vi "LABWAD.vi"() -> ()   [LabVIEW 2017]
uses:
  SubVIs/WAD_MainCluster.ctl
  SubVIs/TextureList.ctl
  SubVIs/PatchList.ctl
  SubVIs/Lumps.ctl
  SubVIs/PLAYPAL.ctl
  Fire/Spread Fire.vi
  <vilib>/picture/picture.llb/Draw 8-Bit Pixmap.vi
  <userlib>/_OpenG.lib/array/array.llb/Filter 1D Array (String)__ogtk.vi
  <userlib>/_OpenG.lib/array/array.llb/Filter 1D Array with Scalar (String)__ogtk.vi
  <vilib>/regexp/Match Regular Expression.xnode
panel:
  out "2D Picture":picture
  in  "File Structure":string[](tree)
  out "Demonic Intensity Graph":i32[][](graph)
  # "Overview: Demonstrates how to read WAD files from original DOOM games.\nRequirements: LabVIEW Full Development System 2017 or compatible\nInstructions:\n1. Run this VI.\n2. Select a .wad file using the File > Open WAD File menu.\n3. Click on different items in the tree view to display them.\n4. Export the displayed image as PNG via drop-down menu on picture, or\n    select and export multiple items from the tree list via drop-down menu.\n5. Quit by using the File > Quit menu."
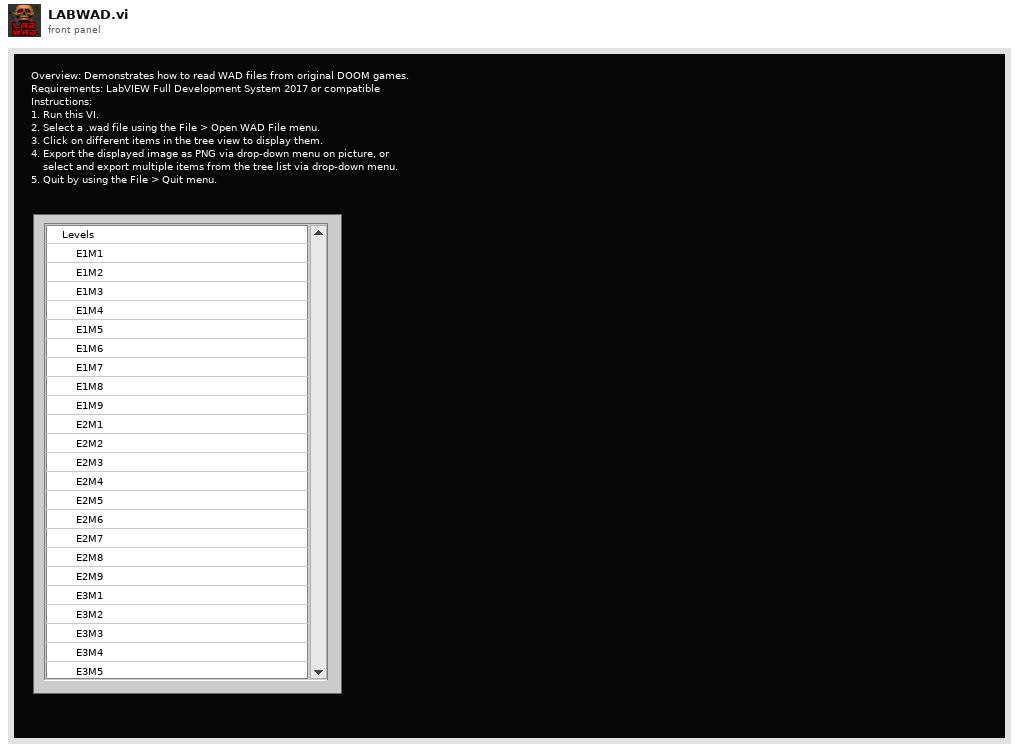
[diagram p1: front panel]
types:
  T1 = typedef "WAD_MainCluster.ctl" = cluster{"WAD file path":path, "WAD as U8 Array":u8[], "WAD Tree":refnum<vi>, "Palette":u32[], "TextureList":T2[], "PNAMES":string[], "Image Array":i16[][], "2D Picture":picture, "Lumps List":string[], "Lumps Array":T4[], "Textures Names":string[], "Image Mask":i16[][], "S_START Index":i32}
  T2 = typedef "TextureList.ctl" = cluster{"Name":string, "flags":u16, "masked":i16, "width":i16, "height":i16, "columndirectory":u32, "patchcount":i16, "PatchList":T3[]}
  T3 = typedef "PatchList.ctl" = cluster{"originx":i16, "originy":i16, "patch":i16}
  T4 = typedef "Lumps.ctl" = cluster{"offData":i32, "lenData":i32, "name":string}
  T5 = typedef "imagedata.ctl" = cluster{"image type":i32, "image depth":i32, "image":u8[], "mask":u8[], "colors":u32[], "Rectangle":cluster{"left":i16, "top":i16, "right":i16, "bottom":i16}}
  T6 = typedef "PatchHeader.ctl" = cluster{"Width":u16, "Height":u16, "XOffset":i16, "YOffset":i16}
  T7 = typedef "PLAYPAL.ctl" = u32[]
  T8 = typedef "LVBoundsTypeDef.ctl" = cluster{"Width":u32, "Height":u32}
  T9 = cluster{"ItemTag":string, "Navigate Tree:Get Path":string[][]}
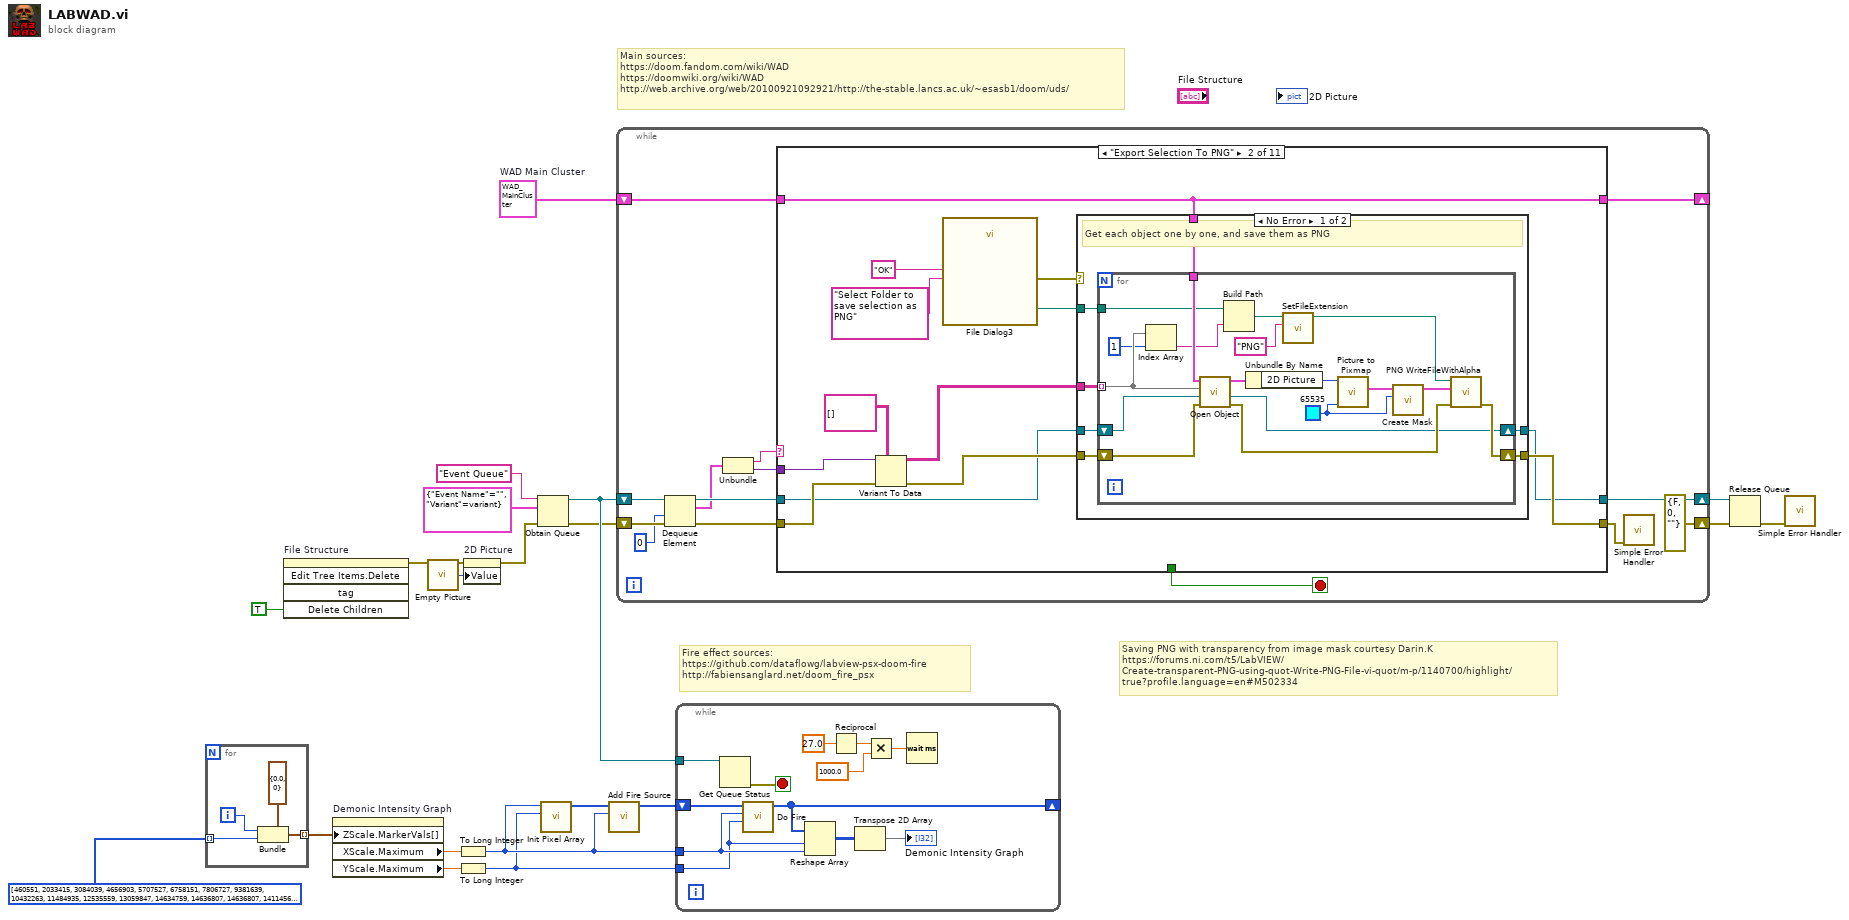
[diagram p0: block diagram]
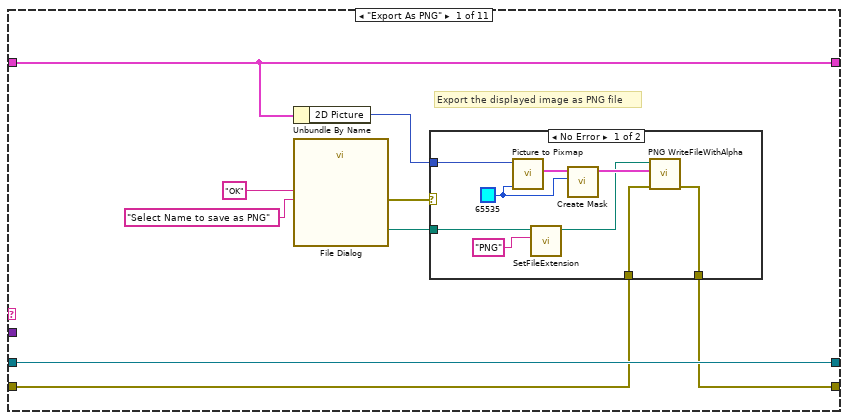
[diagram p2: hidden frame]
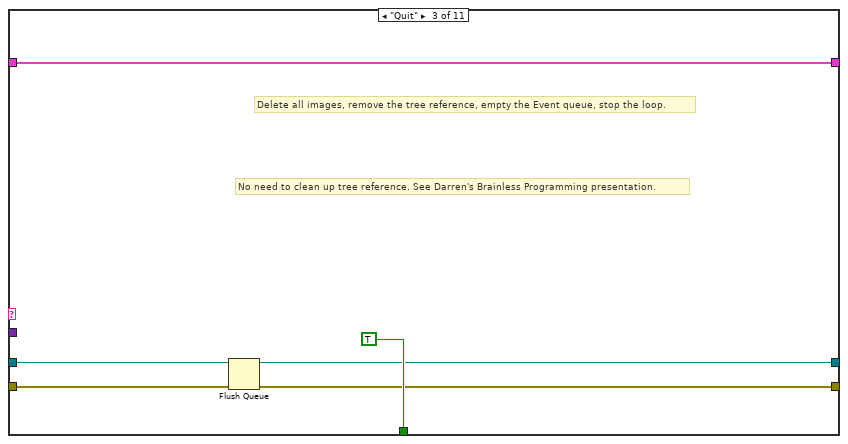
[diagram p5: hidden frame]
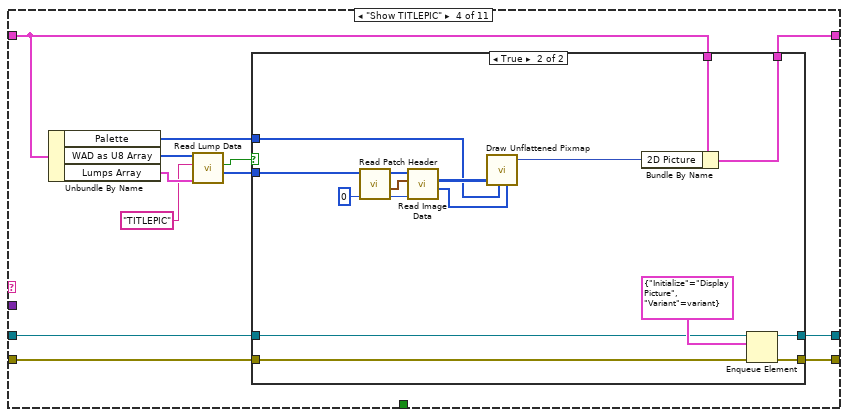
[diagram p6: hidden frame]
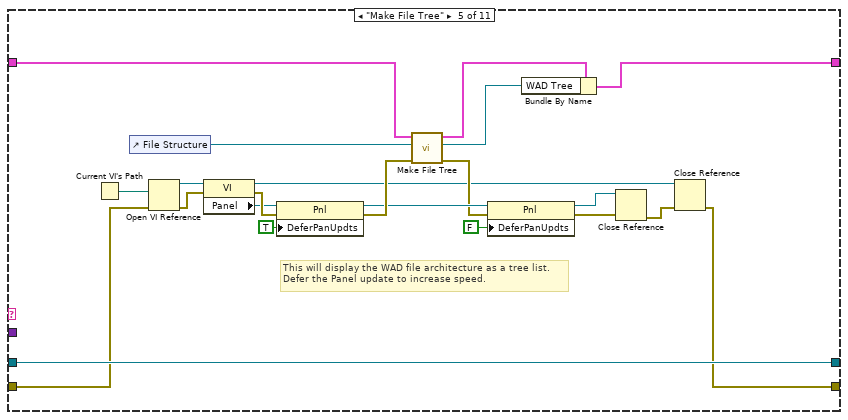
[diagram p8: hidden frame]
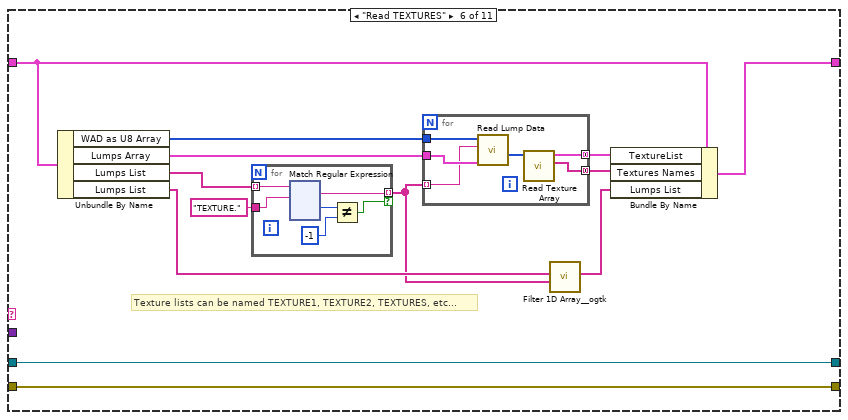
[diagram p9: hidden frame]
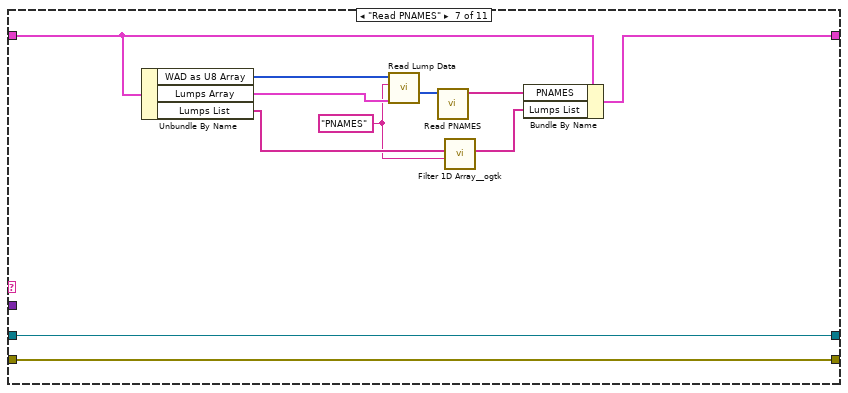
[diagram p10: hidden frame]
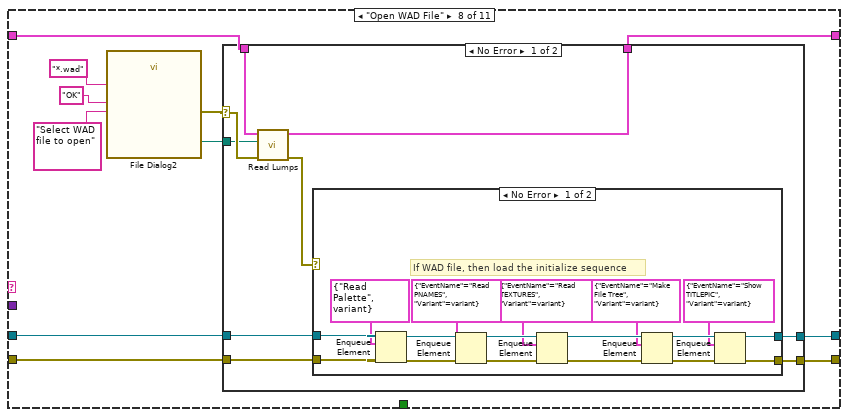
[diagram p11: hidden frame]
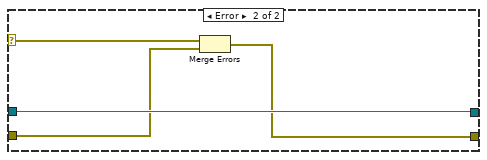
[diagram p12: hidden frame]
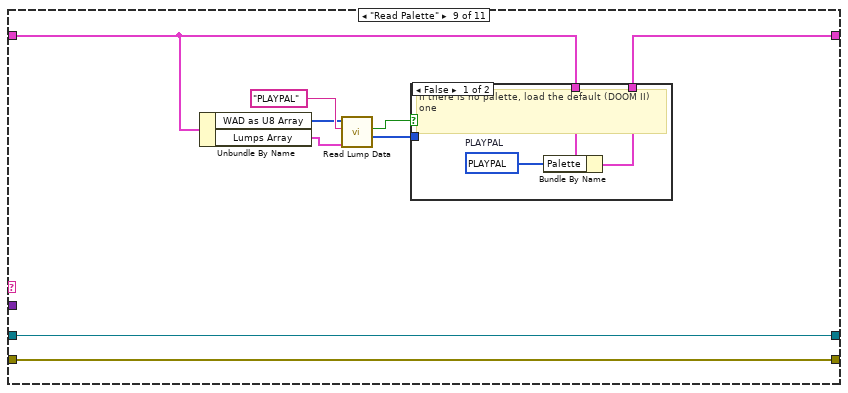
[diagram p14: hidden frame]
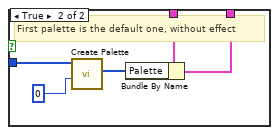
[diagram p15: hidden frame]
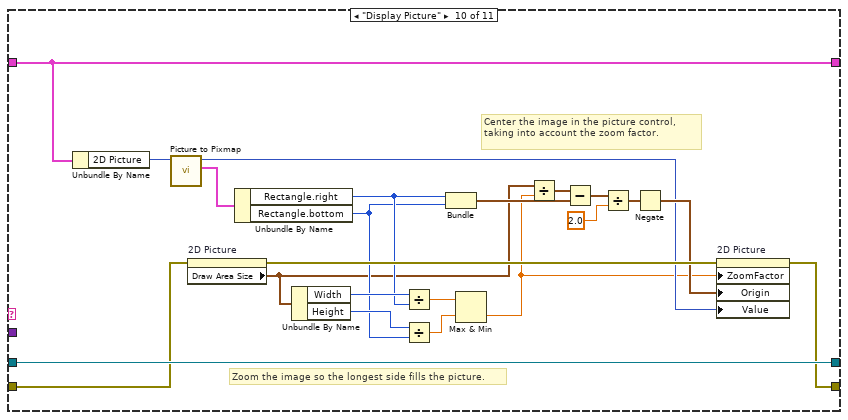
[diagram p16: hidden frame]
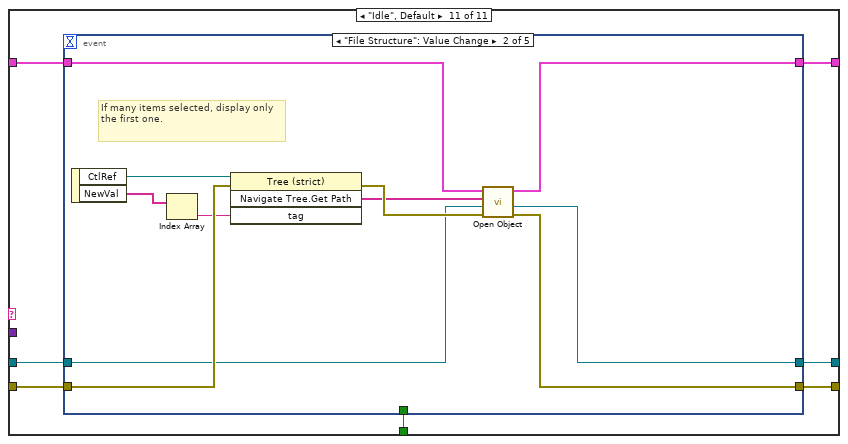
[diagram p17: hidden frame]
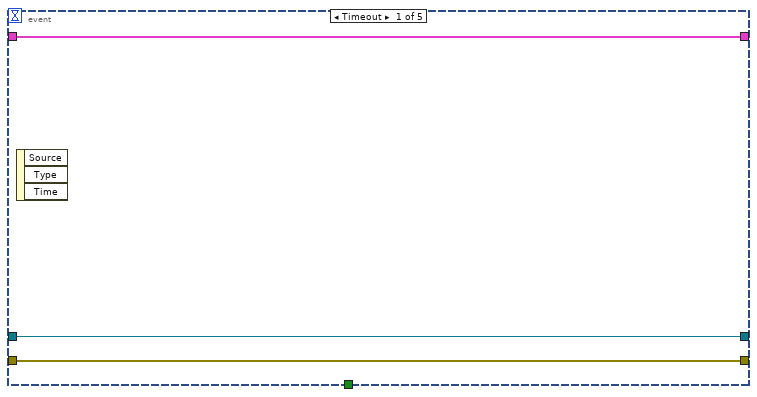
[diagram p18: hidden frame]
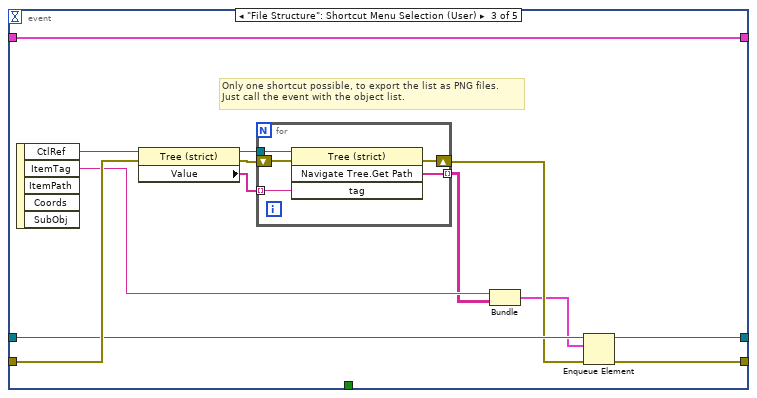
[diagram p19: hidden frame]
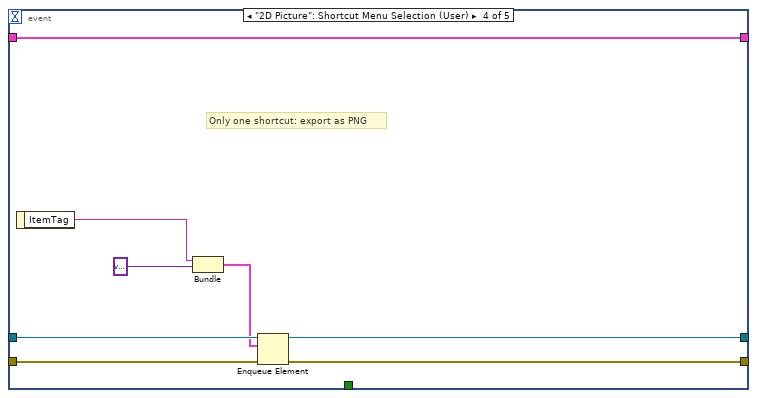
[diagram p20: hidden frame]
diagram:
  w19 = T1 {"WAD file path"=path "", "WAD as U8 Array"=[], "WAD Tree"=refnum, "Palette"=[], "TextureList"=[], "PNAMES"=[], "Image Array"=[], "2D Picture"=bytes[0], "Lumps List"=[], "Lumps Array"=[], "Textures Names"=[], "Image Mask"=[], "S_START Index"=0}  # WAD Main Cluster
  # "Fire effect sources:\nhttps://github.com/dataflowg/labview-psx-doom-fire\nhttp://fabiensanglard.net/doom_fire_psx"
  # "Saving PNG with transparency from image mask courtesy Darin.K\nhttps://forums.ni.com/t5/LabVIEW/Create-transparent-PNG-using-quot-Write-PNG-File-vi-quot/m-p/1140700/highlight/true?profile.language=en#M502334"
  # "Main sources:\nhttps://doom.fandom.com/wiki/WAD\nhttps://doomwiki.org/wiki/WAD\nhttp://web.archive.org/web/20100921092921/http://the-stable.lancs.ac.uk/~esasb1/doom/uds/"
  n1 = for {
    tunnel: u32[] [460551, 2033415, 3084039, 4656903, 5707527, 6758151, 7806727, 9381639, 10432263, 11484935, 12535559, 13059847, 14634759, 14636807, 14636807, 14114567, 14114567, 14116623, 13594383, 13596431, 13598479, 13600535, 13076247, 13078295, 13080351, 12558111, 12558111, 12560167, 12560167, 12562223, 12037935, 12039983, 12039991, 13619055, 14671775, 15724487, 16777215] ("Array") -> [w22] mode=indexing
    tunnel: [w21] -> w6 mode=indexing
    i -> [w23]
    n2 = Bundle(cluster=cluster{dbl, u32} {0.0, 0}, w23, w22) -> (w21:cluster{dbl, u32})
  }
  n3 = invoke on="File Structure" class="Tree (strict)" method="Edit Tree Items.Delete"("Delete Children"=TRUE ("Delete Children?")) -> (error out=w10:errorcluster)  [unwired: 4 in, 4 out]
  n4 = property on="Demonic Intensity Graph" class="IntGraph (strict)"("ZScale.MarkerVals[]"=w6) -> ("XScale.Maximum"=w8:dbl, "YScale.Maximum"=w7:dbl)  [unwired: 2 in, 2 out]
  n5 = call "Empty Picture"() -> ("empty picture"=w11:picture)
  n6 = To Long Integer(number=w8) -> (32bit integer=w5:i32)
  n7 = To Long Integer(number=w7) -> (32bit integer=w4:i32)
  n8 = property on="2D Picture" class="Pict"(error in=w10, "Value"=w11) -> (error out=w9:errorcluster)  [unwired: 1 in, 1 out]
  n9 = Obtain Queue(name (unnamed)="Event Queue", element data type=cluster{"Event Name":string, "Variant":variant} {"Event Name"="", "Variant"=variant}, error in (no error)=w9) -> (queue out=w14:refnum<queue>, error out=w13:errorcluster)  [unwired: 2 in, 1 out]
  n10 = call "Init Pixel Array.vi"("Height"=w4, "Width"=w5) -> ("Pixel Array"=w1:i32[])  [unwired: 9 in]
  n11 = call "Add Fire Source.vi"("Width"=w5, "Pixel Array In"=w1) -> ("Pixel Array Out"=w3:i32[])  [unwired: 9 in]
  n12 = while {
    shift-right: [w37] -> _
    shift-left: w19 -> [w38]
    shift-right: [w36] -> w16
    shift-left: w14 -> [w35]
    shift-right: [errorcluster {"status"=FALSE, "code"=0, "source"=""} ("error out")] -> w17
    shift-left: w13 -> [w34]
    stop <- w28 stop-if-true
    n13 = Dequeue Element(queue=w35, timeout in ms (-1)=0, error in (no error)=w34) -> (queue out=w32:refnum<queue>, element=w31:cluster{"Event Name":string, "Variant":variant}, error out=w33:errorcluster)  [unwired: 1 out]
    n14 = Unbundle(w31) -> ("Event Name"=w30:string, "Variant"=w29:variant)
    n15 = case shown="\"Export Selection To PNG\"" w30 {
      tunnel: w38 -> [w46 w66 w103 w108 w155 w167 w301 w307 w353 w389 w396]
      tunnel: [w46 w66 w103 w107 w135 w166 w299 w317 w352 w389 w395] -> w37
      tunnel: w32 -> [w47 w59 w101 w115 w156 w169 w306 w313 w359 w388 w394]
      tunnel: [w47 w58 w99 w113 w156 w169 w306 w312 w359 w388 w393] -> w36
      tunnel: w33 -> [w39 w67 w100 w114 w147 w168 w305 w309 w358 w379 w392]
      tunnel: [w40 w62 w98 w112 w138 w168 w305 w311 w358 w387 w391] -> w25
      tunnel: w29 -> [_ w70 _ _ _ _ _ _ _ _ _]
      tunnel: [_ _ TRUE _ _ _ _ _ _ _ w390] -> w28
      frame "Export As PNG" {
        # "Export the displayed image as PNG file"
        n16 = Unbundle By Name(w46) -> ("2D Picture"=w45:picture)
        n17 = call "File Dialog"("prompt"="Select Name to save as PNG", "button label"="OK") -> ("selected path"=w42:path, "error out"=w41:errorcluster)  [unwired: 10 in, 2 out]
        n18 = case shown="No Error" w41 {
          tunnel: w45 -> [w51 _]
          tunnel: w42 -> [w56 _]
          tunnel: w39 -> [w49 w57]
          tunnel: [w48 w57] -> w40
          frame No Error {
            w52 = u32 65535 ("Background Color")
            n19 = call <vilib>:"Picture to Pixmap.vi"("Background Color"=w52, "picture"=w51) -> ("image data"=w54:T5)  [unwired: 8 in, 1 out]
            n20 = call "SetFileExtension.vi"("Extension"="PNG" ("button label"), "File path"=w56) -> ("FilePath with Extension"=w50:path)  [unwired: 9 in]
            n21 = call <vilib>:"Create Mask.vi"("Mask Color (Black)"=w52, "image data"=w54) -> ("image data"=w53:T5)  [unwired: 9 in]
            n22 = call "PNG WriteFileWithAlpha.vi"("error in (no error)"=w49, "image data"=w53, "Path to write (dialog)"=w50) -> ("error out"=w48:errorcluster)  [unwired: 7 in, 1 out]
          }
          frame Error {
          }
        }
      }
      frame "Export Selection To PNG" {
        n23 = Variant To Data(error in=w67, type=string[][] [] ("Navigate Tree:Get Path"), Variant=w70) -> (data=w68:string[][], error out=w60:errorcluster)
        n24 = call "File Dialog3"("prompt"="Select Folder to save selection as PNG", "button label"="OK") -> ("selected path"=w63:path, "error out"=w61:errorcluster)  [unwired: 10 in, 2 out]
        n25 = case shown="No Error" w61 {
          tunnel: w68 -> [w77 _]
          tunnel: w60 -> [w76 w97]
          tunnel: w66 -> [w75 _]
          tunnel: w63 -> [w74 _]
          tunnel: [w73 w97] -> w62
          tunnel: w59 -> [w72 w96]
          tunnel: [w71 w96] -> w58
          frame No Error {
            # "Get each object one by one, and save them as PNG"
            n26 = for {
              tunnel: w77 -> [w91] mode=indexing
              shift-right: [w85] -> w73
              shift-left: w76 -> [w94]
              tunnel: w75 -> [w93]
              tunnel: w74 -> [w92]
              shift-right: [w78] -> w71
              shift-left: w72 -> [w79]
              w82 = u32 65535 ("Background Color")
              n27 = Index Array(array=w91, index=1) -> (element=w89:string)
              n28 = call "Open Object.vi"("Error In"=w94, "queue IN"=w79, "Tree Path"=w91, "WAD Cluster IN"=w93) -> ("Error Out"=w86:errorcluster, "queue OUT"=w78:refnum<queue>, "WAD Cluster OUT"=w81:T1)  [unwired: 5 in]
              n29 = Build Path(base path=w92, name or relative path=w89) -> (appended path=w88:path)
              n30 = Unbundle By Name(w81) -> ("2D Picture"=w80:picture)
              n31 = call "SetFileExtension.vi"("Extension"="PNG" ("button label"), "File path"=w88) -> ("FilePath with Extension"=w87:path)  [unwired: 9 in]
              n32 = call <vilib>:"Picture to Pixmap.vi"("Background Color"=w82, "picture"=w80) -> ("image data"=w84:T5)  [unwired: 8 in, 1 out]
              n33 = call <vilib>:"Create Mask.vi"("Mask Color (Black)"=w82, "image data"=w84) -> ("image data"=w83:T5)  [unwired: 9 in]
              n34 = call "PNG WriteFileWithAlpha.vi"("error in (no error)"=w86, "image data"=w83, "Path to write (dialog)"=w87) -> ("error out"=w85:errorcluster)  [unwired: 7 in, 1 out]
            }
          }
          frame Error {
            # "If cancelled, don't do anything"
          }
        }
      }
      frame "Quit" {
        # "No need to clean up tree reference. See Darren's Brainless Programming presentation."
        # "Delete all images, remove the tree reference, empty the Event queue, stop the loop."
        n35 = Flush Queue(queue=w101, error in (no error)=w100) -> (queue out=w99:refnum<queue>, error out=w98:errorcluster)  [unwired: 1 out]
      }
      frame "Show TITLEPIC" {
        n36 = Unbundle By Name(w108) -> ("Palette"=w105:u32[], "WAD as U8 Array"=w111:u8[], "Lumps Array"=w110:T4[])
        n37 = call "Read Lump Data.vi"("Lumps Directory IN"=w110, "Lump Name"="TITLEPIC", "Input U8"=w111) -> ("Lump DATA OUT"=w109:u8[], "Found?"=w106:bool)  [unwired: 5 in, 2 out]
        n38 = case shown="True" w106 {
          tunnel: w115 -> [w117 w133]
          tunnel: w114 -> [w116 w120]
          tunnel: [w117 w132] -> w113
          tunnel: [w116 w131] -> w112
          tunnel: w109 -> [_ w130]
          tunnel: w108 -> [w118 w125]
          tunnel: [w118 w124] -> w107
          tunnel: w105 -> [_ w122]
          frame False {
          }
          frame True {
            n39 = call "Read Patch Header.vi"("Index"=u32 0, "Patch DATA IN"=w130) -> ("Index+8"=w126:u32, "PatchHeader"=w129:T6, "Patch DATA OUT"=w128:u8[])  [unwired: 7 in]
            n40 = call "Read Image Data.vi"("Input Index"=w126, "PatchHeader"=w129, "Patch DATA IN"=w128) -> ("Mask OUT"=w121:u8[], "Image OUT"=w123:u8[][])  [unwired: 5 in, 2 out]
            n41 = call-poly <vilib>:"Draw Unflattened Pixmap.vi"("data"=w123, "color table"=w122, "mask"=w121) -> ("new picture"=w119:picture)  [unwired: 6 in]
            n42 = Bundle By Name(cluster=w125, "2D Picture"=w119) -> (w124:T1)
            n43 = Enqueue Element(queue=w133, element=cluster{"Initialize":string, "Variant":variant} {"Initialize"="Display Picture", "Variant"=variant}, error in (no error)=w120) -> (queue out=w132:refnum<queue>, error out=w131:errorcluster)  [unwired: 1 in, 1 out]
          }
        }
      }
      frame "Make File Tree" {
        # "This will display the WAD file architecture as a tree list.\nDefer the Panel update to increase speed."
        n44 = Current VI's Path() -> (path=w149:path)
        n45 = control-ref of="File Structure"() -> (w154:refnum<vi>)
        n46 = Open VI Reference(vi path=w149, error in (no error)=w147) -> (vi reference=w150:refnum<vi>, error out=w152:errorcluster)  [unwired: 4 in]
        n47 = property class="VI"(reference=w150, error in=w152) -> (reference out=w139:refnum<vi>, error out=w153:errorcluster, "Panel"=w151:refnum<vi>)
        n48 = property class="Pnl"(reference=w151, error in=w153, "DeferPanUpdts"=TRUE ("Defer Panel Updates")) -> (reference out=w144:refnum<vi>, error out=w146:errorcluster)
        n49 = call "Make File Tree.vi"("Error In"=w146, "TreeControl in"=w154, "WAD Main Cluster"=w155) -> ("Error Out"=w143:errorcluster, "TreeControl OUT"=w136:refnum<vi>, "WAD Main Cluster OUT"=w137:T1)  [unwired: 6 in]
        n50 = property class="Pnl"(reference=w144, error in=w143, "DeferPanUpdts"=FALSE ("Defer Panel Updates")) -> (reference out=w141:refnum<vi>, error out=w142:errorcluster)
        n51 = Bundle By Name(cluster=w137, "WAD Tree"=w136) -> (w135:T1)
        n52 = Close Reference(reference=w141, error in (no error)=w142) -> (error out=w140:errorcluster)
        n53 = Close Reference(reference=w139, error in (no error)=w140) -> (error out=w138:errorcluster)
      }
      frame "Read TEXTURES" {
        # "Texture lists can be named TEXTURE1, TEXTURE2, TEXTURES, etc..."
        n54 = Unbundle By Name(w167) -> ("WAD as U8 Array"=w165:u8[], "Lumps Array"=w164:T4[], "Lumps List"=w162:string[], "Lumps List"=w159:string[])
        n55 = for {
          tunnel: w162 -> [w180] mode=indexing
          tunnel: "TEXTURE." ("format string") -> [w181]
          tunnel: [w179] -> w158 mode=indexing if=w176
          n56 = xnode "Match Regular Expression"("input string"=w180, "regular expression"=w181) -> ("whole match"=w179:string, "offset past match"=w178:i32)  [unwired: 4 in, 3 out]
          n57 = Not Equal?(x=w178, y=-1) -> (x != y?=w176:bool)
        }
        n58 = for {
          tunnel: w165 -> [w174]
          tunnel: w164 -> [w173]
          tunnel: [w172] -> w161 mode=concatenating
          tunnel: [w171] -> w160 mode=concatenating
          tunnel: w158 -> [w170] mode=indexing
          n59 = call "Read Lump Data.vi"("Lumps Directory IN"=w173, "Lump Name"=w170, "Input U8"=w174) -> ("Lump DATA OUT"=w175:u8[])  [unwired: 5 in, 3 out]
          n60 = call "Read Texture Array.vi"("TEXTURES Lump"=w175) -> ("Texture Names Array"=w171:string[], "Textures array"=w172:T2[])  [unwired: 9 in]
        }
        n61 = call-poly <userlib>:"Filter 1D Array__ogtk.vi"("items to filter"=w158, "array"=w159) -> ("filtered array"=w157:string[])  [unwired: 4 in, 1 out]
        n62 = Bundle By Name(cluster=w167, "TextureList"=w161, "Textures Names"=w160, "Lumps List"=w157) -> (w166:T1)
      }
      frame "Read PNAMES" {
        w297 = "PNAMES" ("element")
        n63 = Unbundle By Name(w301) -> ("WAD as U8 Array"=w303:u8[], "Lumps Array"=w302:T4[], "Lumps List"=w298:string[])
        n64 = call "Read Lump Data.vi"("Lumps Directory IN"=w302, "Lump Name"=w297, "Input U8"=w303) -> ("Lump DATA OUT"=w304:u8[])  [unwired: 5 in, 3 out]
        n65 = call "Read PNAMES.vi"("Lump DATA IN"=w304) -> ("PNAMES Array"=w300:string[])  [unwired: 10 in]
        n66 = call-poly <userlib>:"Filter 1D Array__ogtk.vi"("items to filter"=w297, "array"=w298) -> ("filtered array"=w296:string[])  [unwired: 4 in, 1 out]
        n67 = Bundle By Name(cluster=w301, "PNAMES"=w300, "Lumps List"=w296) -> (w299:T1)
      }
      frame "Open WAD File" {
        n68 = call "File Dialog2"("prompt"="Select WAD file to open", "button label"="OK", "pattern (all files)"="*.wad") -> ("selected path"=w315:path, "error out"=w310:errorcluster)  [unwired: 9 in, 2 out]
        n69 = case shown="No Error" w310 {
          selector: w310 -> [w321 _]
          tunnel: [w318 w349] -> w317
          tunnel: w315 -> [w320 _]
          tunnel: w313 -> [w326 w350]
          tunnel: w309 -> [w325 w348]
          tunnel: [w324 w350] -> w312
          tunnel: [w323 w348] -> w311
          tunnel: w307 -> [w319 w349]
          frame No Error {
            n70 = call "Read Lumps.vi"("Error In"=w321, "file (use dialog)"=w320, "Cluster"=w319) -> ("Error Out"=w322:errorcluster, "Cluster 2"=w318:T1)  [unwired: 7 in]
            n71 = case shown="No Error" w322 {
              selector: w322 -> [_ w346]
              tunnel: w326 -> [w330 w347]
              tunnel: w325 -> [w329 w345]
              tunnel: [w328 w347] -> w324
              tunnel: [w327 w344] -> w323
              frame No Error {
                # "If WAD file, then load the initialize sequence"
                n72 = Enqueue Element(queue=w330, element=cluster{"EventName":string, "Variant":variant} {"EventName"="Read Palette", "Variant"=variant}, error in (no error)=w329) -> (queue out=w341:refnum<queue>, error out=w340:errorcluster)  [unwired: 1 in, 1 out]
                n73 = Enqueue Element(queue=w341, element=cluster{"EventName":string, "Variant":variant} {"EventName"="Read PNAMES", "Variant"=variant}, error in (no error)=w340) -> (queue out=w343:refnum<queue>, error out=w342:errorcluster)  [unwired: 1 in, 1 out]
                n74 = Enqueue Element(queue=w343, element=cluster{"EventName":string, "Variant":variant} {"EventName"="Read TEXTURES", "Variant"=variant}, error in (no error)=w342) -> (queue out=w337:refnum<queue>, error out=w336:errorcluster)  [unwired: 1 in, 1 out]
                n75 = Enqueue Element(queue=w337, element=cluster{"EventName":string, "Variant":variant} {"EventName"="Make File Tree", "Variant"=variant}, error in (no error)=w336) -> (queue out=w339:refnum<queue>, error out=w338:errorcluster)  [unwired: 1 in, 1 out]
                n76 = Enqueue Element(queue=w339, element=cluster{"EventName":string, "Variant":variant} {"EventName"="Show TITLEPIC", "Variant"=variant}, error in (no error)=w338) -> (queue out=w328:refnum<queue>, error out=w327:errorcluster)  [unwired: 1 in, 1 out]
              }
              frame Error {
                n77 = Merge Errors(w346, w345) -> (w344:errorcluster)
              }
            }
          }
          frame Error {
          }
        }
      }
      frame "Read Palette" {
        n78 = Unbundle By Name(w353) -> ("WAD as U8 Array"=w356:u8[], "Lumps Array"=w355:T4[])
        n79 = call "Read Lump Data.vi"("Lumps Directory IN"=w355, "Lump Name"="PLAYPAL" ("element"), "Input U8"=w356) -> ("Lump DATA OUT"=w354:u8[], "Found?"=w351:bool)  [unwired: 5 in, 2 out]
        n80 = case shown="False" w351 {
          tunnel: w354 -> [_ w366]
          tunnel: w353 -> [w362 w365]
          tunnel: [w361 w363] -> w352
          frame False {
            w360 = T7 [0, 2037515, 1511175, 4934475, 16777215, 1776411, 1250067, 723723, 460551, 3094303, 2304783, 1515271, 988928, 5192491, 4666147, 4139803, 16758711, 16231339, 15967139, 15439767, 15175567, 14649223, 14383995, 13857651, 13331307, 13067107, 12540763, 12277591, 11751247, 11487047, 10960703, 10697531, 10171187, 9908015, 9382699, 9118499, 8593183, 8330011, 7804695, 7541523, 7016207, 6753035, 6227719, 5965575, 5441287, 5177344, 4653056, 4390912, 16772063, 16770003, 16767943, 16765883, 16764851, 16762791, 16760731, 16759699, 16757635, 16231291, 15704947, 15178603, 14652259, 14125915, 13599571, 13336399, 12548939, 11760455, 11235139, 10709823, 10183483, 9396023, 8869683, 8344367, 7819051, 7030567, 6243107, 5455647, 4929307, 4140823, 3353363, 2827023, 15724527, 15198183, 14671839, 14408667, 13882323, 13355979, 13092807, 12566463, 12040119, 11776947, 11250603, 10987431, 10461087, 9934743, 9671571, 9145227, 8618883, 8355711, 7829367, 7303023, 7039851, 6513507, 5987163, 5723991, 5197647, 4671303, 4408131, 3881787, 3618615, 3092271, 2565927, 2302755, 7864175, 7335783, 6807391, 6278999, 6012751, 5484359, 4955967, 4428599, 4162351, 3633963, 3105571, 2577179, 2048791, 1520399, 1254155, 726791, 12560271, 12033927, 11507583, 10981239, 10454895, 10190699, 9665379, 9139035, 8612695, 8086351, 7823179, 7296835, 6771519, 6245175, 5718835, 5455663, 10453859, 9402195, 8612683, 7823167, 6771507, 5981995, 5192483, 4403995, 8093539, 7304023, 6777679, 5989191, 5461819, 4673331, 4146987, 3620647, 16777075, 15457111, 14138179, 12819247, 11500319, 10181395, 8864519, 7547648, 16777215, 16767963, 16759739, 16751515, 16743291, 16736095, 16727871, 16719647, 16711680, 15663104, 14876672, 14090240, 13303808, 12517376, 11730944, 10944512, 10158080, 9109504, 8323072, 7536640, 6750208, 5963776, 5177344, 4390912, 15198207, 13092863, 11250687, 9408511, 7566335, 5460991, 3618815, 1776639, 255, 227, 203, 179, 155, 131, 107, 83, 16777215, 16772059, 16766907, 16762779, 16757627, 16753499, 16748347, 16744219, 15954711, 15429391, 14640911, 14114571, 13326087, 12799744, 12011264, 11485952, 16777215, 16777175, 16777139, 16777103, 16777067, 16777031, 16776995, 16776960, 10960640, 10434304, 9645824, 8856320, 5192487, 4402971, 3613459, 3087115, 83, 71, 59, 47, 35, 23, 11, 0, 16752451, 16770891, 16743423, 16711935, 13566159, 10420379, 7274603, 10972011]  # PLAYPAL
            # "If there is no palette, load the default (DOOM II) one"
            n81 = Bundle By Name(cluster=w362, "Palette"=w360) -> (w361:T1)
          }
          frame True {
            # "First palette is the default one, without effect"
            n82 = call "Create Palette.vi"("Palette Index"=0 ("index"), "Palette Lump"=w366) -> ("Palette"=w364:u32[])  [unwired: 9 in]
            n83 = Bundle By Name(cluster=w365, "Palette"=w364) -> (w363:T1)
          }
        }
      }
      frame "Display Picture" {
        # "Center the image in the picture control, taking into account the zoom factor."
        # "Zoom the image so the longest side fills the picture."
        n84 = Unbundle By Name(w389) -> ("2D Picture"=w386:picture)
        n85 = call <vilib>:"Picture to Pixmap.vi"("picture"=w386) -> ("image data"=w385:T5, "new picture"=w370:picture)  [unwired: 9 in]
        n86 = property on="2D Picture" class="Pict"(error in=w379) -> (error out=w380:errorcluster, "Draw Area Size"=w368:T8)  [unwired: 1 in, 1 out]
        n87 = Unbundle By Name(w385) -> ("Rectangle.right"=w377:i16, "Rectangle.bottom"=w376:i16)
        n88 = Unbundle By Name(w368) -> ("Width"=w384:u32, "Height"=w383:u32)
        n89 = Divide(x=w384, y=w377) -> (x/y=w382:dbl)
        n90 = Divide(x=w383, y=w376) -> (x/y=w381:dbl)
        n91 = Bundle("right"=w377, "bottom"=w376) -> (w375:cluster{"right":i16, "bottom":i16})  [unwired: 1 in]
        n92 = Max & Min(x=w382, y=w381) -> (min(x,y)=w369:dbl)  [unwired: 1 out]
        n93 = Divide(x=w368, y=w369) -> (x/y=w378:cluster{"Width":dbl, "Height":dbl})
        n94 = Subtract(x=w378, y=w375) -> (x-y=w374:cluster{dbl, dbl})
        n95 = Divide(x=w374, y=2.0) -> (x/y=w372:cluster{dbl, dbl})
        n96 = Negate(x=w372) -> (-x=w371:cluster{dbl, dbl})
        n97 = property on="2D Picture" class="Pict"(error in=w380, "ZoomFactor"=w369, "Origin"=w371, "Value"=w370) -> (error out=w387:errorcluster)  [unwired: 1 in, 1 out]
      }
      frame "Idle", Default {
        n98 = event shown="[1] \"File Structure\": Value Change" {
          selector: _ -> [_ _ _ _ _]
          dyn-events: _ -> [_ _ _ _ _]
          timeout: _ -> [_ _ _ _ _]
          tunnel: w396 -> [w399 w408 w418 w436 w445]
          tunnel: [w399 w403 w418 w436 w445] -> w395
          tunnel: w394 -> [w398 w402 w417 w435 w444]
          tunnel: [w398 w400 w415 w433 w442] -> w393
          tunnel: w392 -> [w397 w406 w422 w434 w443]
          tunnel: [w397 w401 w414 w432 w441] -> w391
          tunnel: [_ _ _ _ FALSE] -> w390
          event Timeout {
            n99 = event-data() -> ()  [unwired: 1 in, 3 out]
          }
          event "File Structure": Value Change {
            # "If many items selected, display only the first one."
            n100 = event-data() -> ("CtlRef"=w407:refnum<vi>, "NewVal"=w405:string[])  [unwired: 1 in]
            n101 = Index Array(array=w405) -> (element=w404:string)  [unwired: 1 in]
            n102 = invoke class="Tree (strict)" method="Navigate Tree.Get Path"(reference=w407, error in=w406, "tag"=w404) -> (error out=w410:errorcluster, "Navigate Tree:Get Path"=w409:string[])  [unwired: 1 in, 2 out]
            n103 = call "Open Object.vi"("Error In"=w410, "queue IN"=w402, "Tree Path"=w409, "WAD Cluster IN"=w408) -> ("Error Out"=w401:errorcluster, "queue OUT"=w400:refnum<queue>, "WAD Cluster OUT"=w403:T1)  [unwired: 5 in]
          }
          event "File Structure": Shortcut Menu Selection (User) {
            # "Only one shortcut possible, to export the list as PNG files.\nJust call the event with the object list."
            n104 = event-data() -> ("CtlRef"=w423:refnum<vi>, "ItemTag"=w413:string)  [unwired: 1 in, 3 out]
            n105 = property class="Tree (strict)"(reference=w423, error in=w422) -> (reference out=w421:refnum<vi>, error out=w420:errorcluster, "Value"=w419:string[])
            n106 = for {
              tunnel: w421 -> [w428]
              tunnel: w419 -> [w426] mode=indexing
              shift-right: [w425] -> w416
              shift-left: w420 -> [w427]
              tunnel: [w424] -> w412 mode=indexing
              n107 = invoke class="Tree (strict)" method="Navigate Tree.Get Path"(reference=w428, error in=w427, "tag"=w426) -> (error out=w425:errorcluster, "Navigate Tree:Get Path"=w424:string[])  [unwired: 1 in, 2 out]
            }
            n108 = Bundle("ItemTag"=w413, "Navigate Tree:Get Path"=w412) -> (w411:T9)  [unwired: 1 in]
            n109 = Enqueue Element(queue=w417, element=w411, error in (no error)=w416) -> (queue out=w415:refnum<queue>, error out=w414:errorcluster)  [unwired: 1 in, 1 out]
          }
          event "2D Picture": Shortcut Menu Selection (User) {
            # "Only one shortcut: export as PNG"
            n110 = event-data() -> ("ItemTag"=w431:string)  [unwired: 1 in]
            n111 = Bundle("ItemTag"=w431, "Variant"=variant) -> (w429:cluster{"ItemTag":string, "Variant":variant})  [unwired: 1 in]
            n112 = Enqueue Element(queue=w435, element=w429, error in (no error)=w434) -> (queue out=w433:refnum<queue>, error out=w432:errorcluster)  [unwired: 1 in, 1 out]
          }
          event Menu Selection (User) {
            n113 = event-data() -> ("ItemTag"=w440:string)  [unwired: 1 in]
            n114 = Bundle("ItemTag"=w440, "Variant"=variant) -> (w438:cluster{"ItemTag":string, "Variant":variant})  [unwired: 1 in]
            n115 = Enqueue Element(queue=w444, element=w438, error in (no error)=w443) -> (queue out=w442:refnum<queue>, error out=w441:errorcluster)  [unwired: 1 in, 1 out]
          }
        }
      }
    }
    n116 = call <vilib>:"Simple Error Handler.vi"("error in (no error)"=w25) -> ()  [unwired: 4 in, 5 out]
  }
  n117 = while {
    shift-right: [w452] -> _
    shift-left: w3 -> [w446]
    tunnel: w5 -> [w451]
    tunnel: w4 -> [w450]
    tunnel: w14 -> [w449]
    stop <- w448 stop-if-true
    n118 = Get Queue Status(queue=w449) -> (error out=w448:errorcluster)  [unwired: 2 in, 7 out]
    n119 = call "Do Fire.vi"("Height"=w450, "Width"=w451, "Pixel Array In"=w446) -> ("Pixel Array Out"=w452:i32[])  [unwired: 8 in]
    n120 = Reshape Array(w452, w450, w451) -> (w454:i32[][])
    n121 = Reciprocal(x=27.0) -> (1/x=w457:dbl)
    n122 = Transpose 2D Array(2D array=w454) -> (transposed array=→"Demonic Intensity Graph":i32[][])
    n123 = Multiply(x=w457, y=1000.0) -> (x*y=w455:dbl)
    n124 = Wait (ms)(milliseconds to wait=w455) -> ()  [unwired: 1 out]
  }
  n125 = Release Queue(queue=w16, error in (no error)=w17) -> (error out=w15:errorcluster)  [unwired: 1 in, 2 out]
  n126 = call <vilib>:"Simple Error Handler.vi"("error in (no error)"=w15) -> ()  [unwired: 4 in, 5 out]
